vi "Write NumAvg.vi"(8 "error in (no error)":errorcluster, 10 "NumAvg":u32=1 caption="Number of averages", 11 "SEDSpectrometer in":refnum<class "SEDSpectrometer.lvclass">) -> (0 "error out":errorcluster, 3 "SEDSpectrometer out":refnum<class "SEDSpectrometer.lvclass">)   [LabVIEW 2016, in "SEDSpectrometer.lvclass"]
uses:
  SEDSpectrometer.lvclass
  SEDSpectrometer.lvclass/SEDSpectrometer.ctl
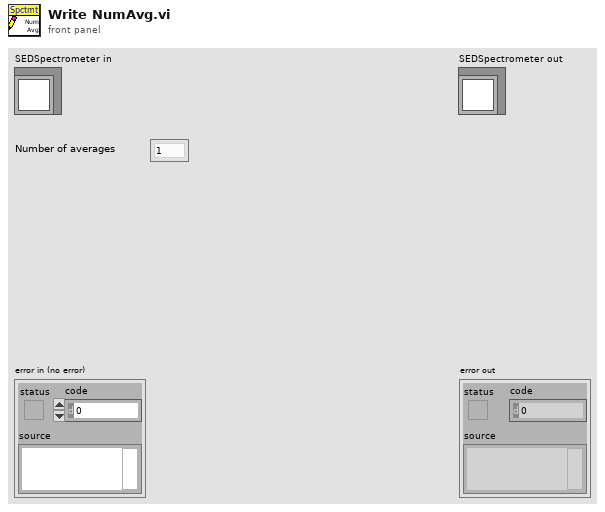
[diagram p1: front panel]
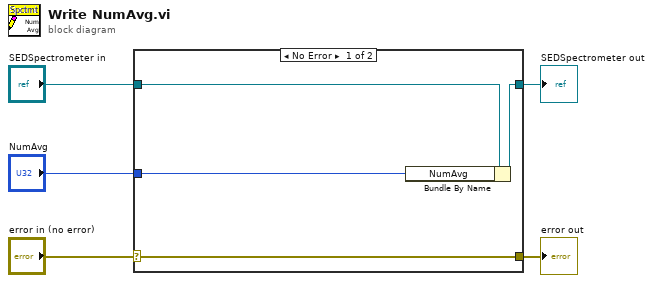
[diagram p0: block diagram]
diagram:
  n1 = case shown="No Error" "error in (no error)" {
    selector: "error in (no error)" -> [w9 w10]
    tunnel: [w9 w10] -> w4
    tunnel: [w7 w11] -> w2
    tunnel: "SEDSpectrometer in" -> [w8 w11]
    tunnel: "NumAvg" -> [w6 _]
    frame No Error {
      n2 = Bundle By Name(cluster=w8, "NumAvg"=w6) -> (w7:refnum<class "SEDSpectrometer.lvclass">)
    }
    frame Error {
    }
  }
  "error out" <- w4
  "SEDSpectrometer out" <- w2
